vi "Directory to Files.vi"(3 "error in":errorcluster, 5 "Directory Path":path[](array[path])) -> (0 "error out":errorcluster, 1 "Cover Files":path[](array[path]), 2 "Music Files":path[](array[path]))   [LabVIEW 2024]
panel:
  # "Connector Pane"
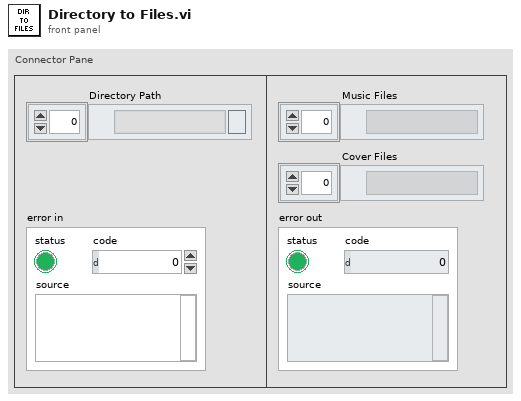
[diagram p1: front panel]
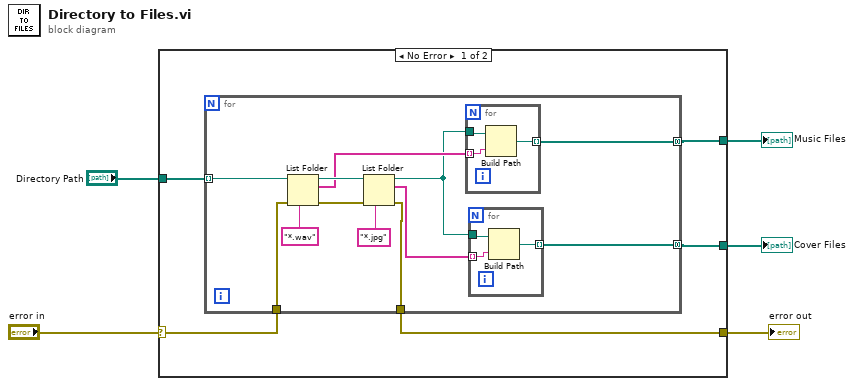
[diagram p0: block diagram]
diagram:
  n1 = case shown="No Error" "error in" {
    selector: "error in" -> [w6 w29]
    tunnel: "Directory Path" -> [w10 _]
    tunnel: [w7 w29] -> w3
    tunnel: [w9 _] -> w2
    tunnel: [w8 _] -> w1
    frame No Error {
      n2 = for {
        tunnel: w10 -> [w18] mode=indexing
        tunnel: [w14] -> w9 mode=concatenating
        tunnel: [w13] -> w8 mode=concatenating
        tunnel: [w12] -> w7
        tunnel: w6 -> [w11]
        n3 = List Folder(path=w18, pattern="*.wav", error in=w11) -> (path out=w22:path, filenames=w17:string[], error out=w21:errorcluster)  [unwired: 1 in, 1 out]
        n4 = List Folder(path=w22, pattern="*.jpg", error in=w21) -> (path out=w15:path, filenames=w16:string[], error out=w12:errorcluster)  [unwired: 1 in, 1 out]
        n5 = for {
          tunnel: w17 -> [w28] mode=indexing
          tunnel: w15 -> [w26]
          tunnel: [w27] -> w14 mode=indexing
          n6 = Build Path(base path=w26, name or relative path=w28) -> (appended path=w27:path)
        }
        n7 = for {
          tunnel: w16 -> [w25] mode=indexing
          tunnel: w15 -> [w23]
          tunnel: [w24] -> w13 mode=indexing
          n8 = Build Path(base path=w23, name or relative path=w25) -> (appended path=w24:path)
        }
      }
    }
    frame Error {
    }
  }
  "error out" <- w3
  "Music Files" <- w2
  "Cover Files" <- w1
